vi "subin_160607_85.vi"() -> ()   [LabVIEW 2015]
uses:
  <vilib>/NXT/Block Support/NXT_OutputPort.ctl
  <vilib>/NXT/Block Support/NXT_InputPort.ctl
  <vilib>/NXT/NXTIO Xnodes/NXTIONodeSubVIs/NXTMoveMotors.vi
  <vilib>/NXT/Dual Mode Library/Waits/Wait_Num.vi
  <vilib>/NXT/Dual Mode Library/Sensors/Light_On.vi
  <vilib>/NXT/Dual Mode Library/Sensors/Touch_Pressed.vi
  <vilib>/NXT/Dual Mode Library/Sensors/Sonar_cm.vi
  <vilib>/NXT/NXTIO Xnodes/AddressXNode/NXTIOAddress.xnode
  <vilib>/NXT/Subs/LVHSConnector.ctl
  <vilib>/NXT/NXTIO Xnodes/NXTIOXNode/NXTIO.xnode
  <vilib>/NXT/LegoClasses/BrickReference/BrickReference.lvclass
panel:
  in  "start C":i8=75
  in  "bouble white left turn C":i8=75
  in  "bouble white left turn B":i8=75
  in  "start B":i8=75
  in  "turn lefttC 2":i8=75
  in  "turn lefttB 2":i8=75
  in  "Go-ahead":i8=75
  out "check destance":i16(slide) scale=0.0..100.0
  in  "turn rightC":i8=75
  in  "turn rightB":i8=75
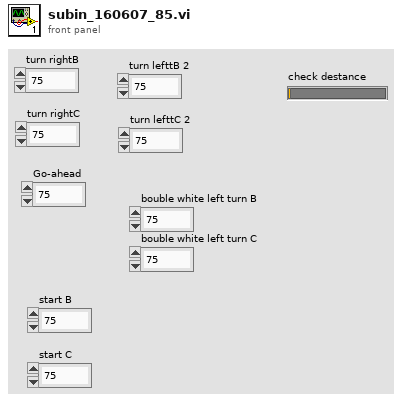
[diagram p1: front panel]
types:
  T1 = typedef "NXT_OutputPort.ctl" = u8
  T2 = typedef "LVHSConnector.ctl" = refnum<class "BrickReference.lvclass">
  T3 = typedef "NXT_InputPort.ctl" = u32
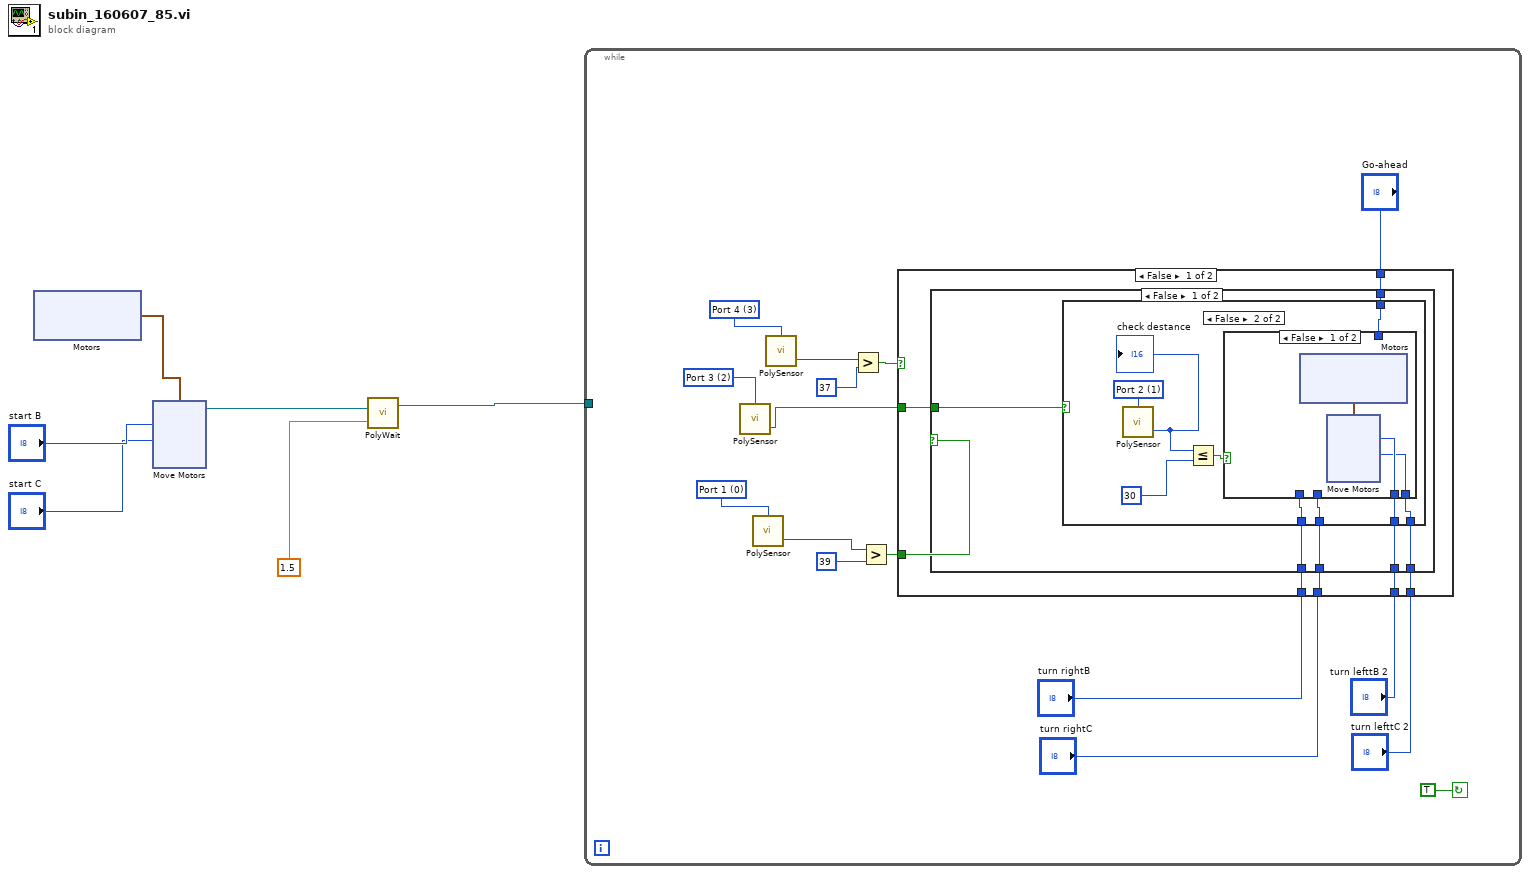
[diagram p0: block diagram]
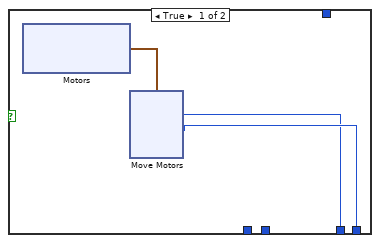
[diagram p2: hidden frame]
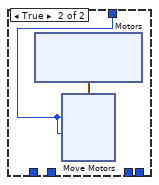
[diagram p3: hidden frame]
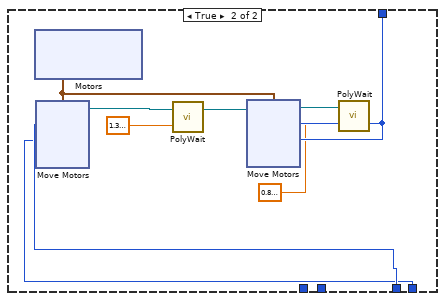
[diagram p4: hidden frame]
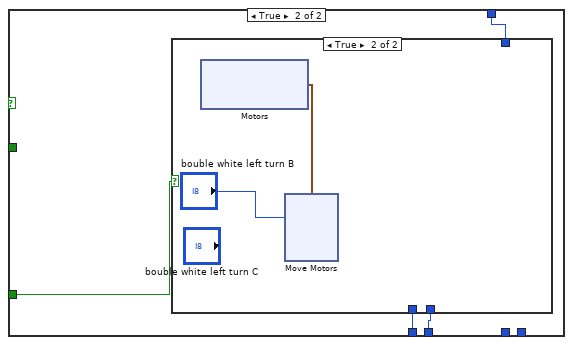
[diagram p5: hidden frame]
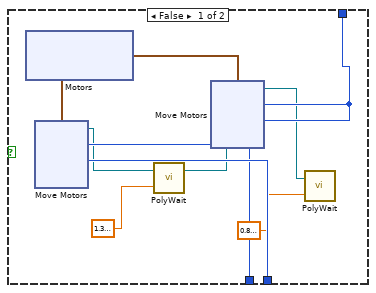
[diagram p6: hidden frame]
diagram:
  n1 = xnode "Motors"() -> ("Motor"=w6:cluster{"Port":T1, "Port":T1})
  n2 = xnode "Move Motors"("Power/Speed 1"="start B", "Motors"=w6, "Power/Speed 2"="start C") -> ("NXT/EV3"=w5:T2)  [unwired: 1 in]
  n3 = call-poly <vilib>:"PolyWait.vi"("Time (1 sec)"=sgl 1.5, "NXT/EV3"=w5) -> ("NXT/EV3"=w4:T2)  [unwired: 2 in]
  n4 = while {
    tunnel: w4 -> [_]
    stop <- TRUE continue-if-true
    w7 = T3 2 items=["Port 1", "Port 2", "Port 3", "Port 4"] ("Port (Port 1)")
    w18 = T3 3 items=["Port 1", "Port 2", "Port 3", "Port 4"] ("Port (Port 3)")
    w17 = T3 0 items=["Port 1", "Port 2", "Port 3", "Port 4"] ("Port (Port 3)")
    n5 = call-poly <vilib>:"PolySensor.vi"("Port (Port 1)"=w7) -> ("Yes / No"=w8:bool)  [unwired: 2 in, 1 out]
    n6 = call-poly <vilib>:"PolySensor.vi"("Port (Port 3)"=w17) -> ("Scaled Value"=w19:i16)  [unwired: 2 in, 1 out]
    n7 = call-poly <vilib>:"PolySensor.vi"("Port (Port 3)"=w18) -> ("Scaled Value"=w21:i16)  [unwired: 2 in, 1 out]
    n8 = Greater?(x=w21, y=i16 37) -> (0:w16:bool)
    n9 = Greater?(x=w19, y=i16 39) -> (0:w15:bool)
    n10 = case shown="False" w16 {
      tunnel: w15 -> [w29 w109]
      tunnel: "turn rightB" -> [w28 w108]
      tunnel: "turn rightC" -> [w27 w107]
      tunnel: "Go-ahead" -> [w26 w106]
      tunnel: "turn lefttB 2" -> [w25 _]
      tunnel: "turn lefttC 2" -> [w24 _]
      tunnel: w8 -> [w23 _]
      frame False {
        n11 = case shown="False" w29 {
          tunnel: w28 -> [w35 _]
          tunnel: w27 -> [w34 _]
          tunnel: w26 -> [w33 w84]
          tunnel: w25 -> [w31 w88]
          tunnel: w24 -> [w30 w87]
          tunnel: w23 -> [w32 _]
          frame False {
            n12 = case shown="False" w32 {
              tunnel: w35 -> [_ w56]
              tunnel: w34 -> [_ w55]
              tunnel: w33 -> [_ w50]
              tunnel: w31 -> [w36 w49]
              tunnel: w30 -> [w37 w48]
              frame True {
                n13 = xnode "Motors"() -> ("Motor"=w38:cluster{"Port":T1, "Port":T1})
                n14 = xnode "Move Motors"("Power/Speed 2"=w37, "Power/Speed 1"=w36, "Motors"=w38) -> ()  [unwired: 1 in, 1 out]
              }
              frame False {
                w53 = T3 1 items=["Port 1", "Port 2", "Port 3", "Port 4"] ("Port (Port 4)")
                n15 = call-poly <vilib>:"PolySensor.vi"("Port (Port 4)"=w53) -> ("Distance (cm)"=w54:i16)  [unwired: 2 in, 1 out]
                "check destance" <- w54
                n16 = Less Or Equal?(x=w54, y=i16 30) -> (x <= y?=w51:bool)
                n17 = case shown="False" w51 {
                  tunnel: w56 -> [_ _]
                  tunnel: w55 -> [_ _]
                  tunnel: w50 -> [_ w69]
                  tunnel: w49 -> [w58 _]
                  tunnel: w48 -> [w57 _]
                  frame False {
                    n18 = xnode "Motors"() -> ("Motor"=w59:cluster{"Port":T1, "Port":T1})
                    n19 = xnode "Move Motors"("Power/Speed 2"=w57, "Power/Speed 1"=w58, "Motors"=w59) -> ()  [unwired: 1 in, 1 out]
                  }
                  frame True {
                    n20 = xnode "Motors"() -> ("Motor"=w70:cluster{"Port":T1, "Port":T1})
                    n21 = xnode "Move Motors"("Power/Speed 2"=w69, "Power/Speed 1"=w69, "Motors"=w70) -> ()  [unwired: 1 in, 1 out]
                  }
                }
              }
            }
          }
          frame True {
            n22 = xnode "Motors"() -> ("Motor"=w85:cluster{"Port":T1, "Port":T1})
            n23 = xnode "Move Motors"("Power/Speed 2"=w87, "Power/Speed 1"=w88, "Motors"=w85) -> ("NXT/EV3"=w86:T2)  [unwired: 1 in]
            n24 = call-poly <vilib>:"PolyWait.vi"("Time (1 sec)"=sgl 1.4, "NXT/EV3"=w86) -> ("NXT/EV3"=w83:T2)  [unwired: 2 in]
            n25 = xnode "Move Motors"("Power/Speed 2"=w84, "Power/Speed 1"=w84, "Motors"=w85, "NXT/EV3"=w83) -> ("NXT/EV3"=w82:T2)
            n26 = call-poly <vilib>:"PolyWait.vi"("Time (1 sec)"=sgl 0.8, "NXT/EV3"=w82) -> ()  [unwired: 2 in, 1 out]
          }
        }
      }
      frame True {
        n27 = case shown="True" w109 {
          tunnel: w108 -> [w117 _]
          tunnel: w107 -> [w118 _]
          tunnel: w106 -> [w115 _]
          frame False {
            n28 = xnode "Motors"() -> ("Motor"=w116:cluster{"Port":T1, "Port":T1})
            n29 = xnode "Move Motors"("Power/Speed 2"=w118, "Power/Speed 1"=w117, "Motors"=w116) -> ("NXT/EV3"=w114:T2)  [unwired: 1 in]
            n30 = call-poly <vilib>:"PolyWait.vi"("Time (1 sec)"=sgl 1.4, "NXT/EV3"=w114) -> ("NXT/EV3"=w113:T2)  [unwired: 2 in]
            n31 = xnode "Move Motors"("Power/Speed 2"=w115, "Power/Speed 1"=w115, "Motors"=w116, "NXT/EV3"=w113) -> ("NXT/EV3"=w112:T2)
            n32 = call-poly <vilib>:"PolyWait.vi"("Time (1 sec)"=sgl 0.8, "NXT/EV3"=w112) -> ()  [unwired: 2 in, 1 out]
          }
          frame True {
            n33 = xnode "Motors"() -> ("Motor"=w137:cluster{"Port":T1, "Port":T1})
            n34 = xnode "Move Motors"("Power/Speed 1"="bouble white left turn B", "Motors"=w137) -> ()  [unwired: 2 in, 1 out]
          }
        }
      }
    }
  }
